vi "Process Depth.vi"(8 "Height":i32=480, 9 "Width":i32=640, 10 "Depth Format":u16(ring)=3 items=["11 Bit", "10 Bit", "11 Bit (Packed)", "10 Bit (Packed)"]) -> (3 "Depth Reshape Array":u16[][](array[numeric]))   [LabVIEW 2012]
panel:
  out "error out":errorcluster
  in  "error in":errorcluster
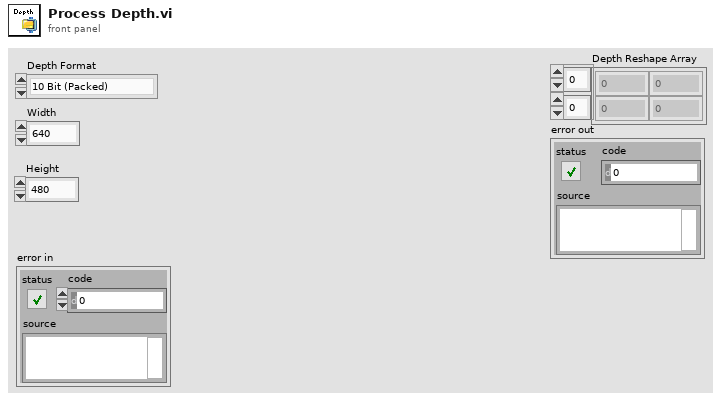
[diagram p1: front panel]
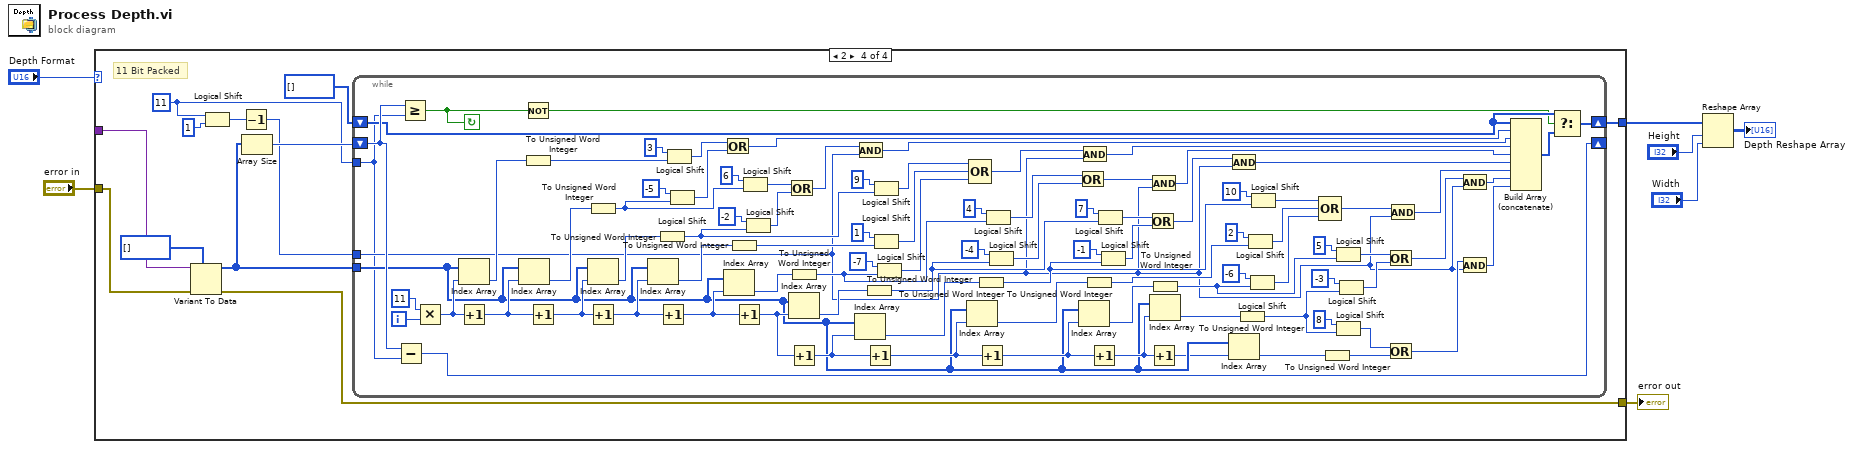
[diagram p0: block diagram]
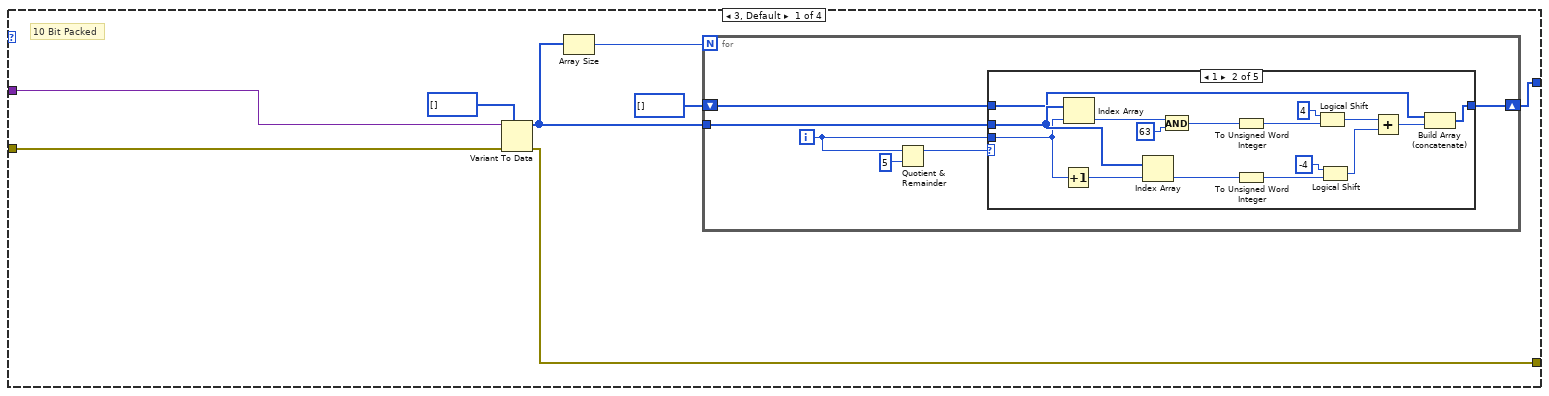
[diagram p2: hidden frame]
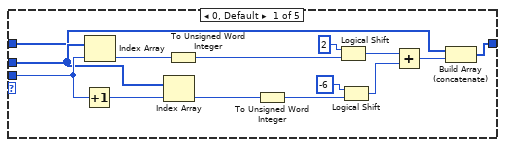
[diagram p3: hidden frame]
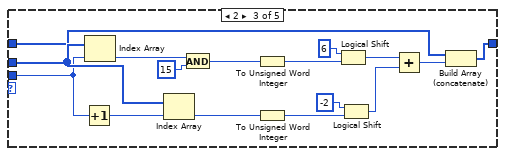
[diagram p4: hidden frame]
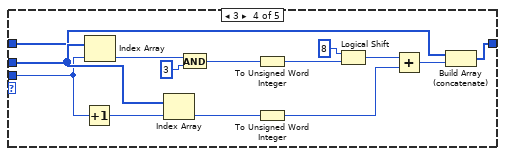
[diagram p5: hidden frame]
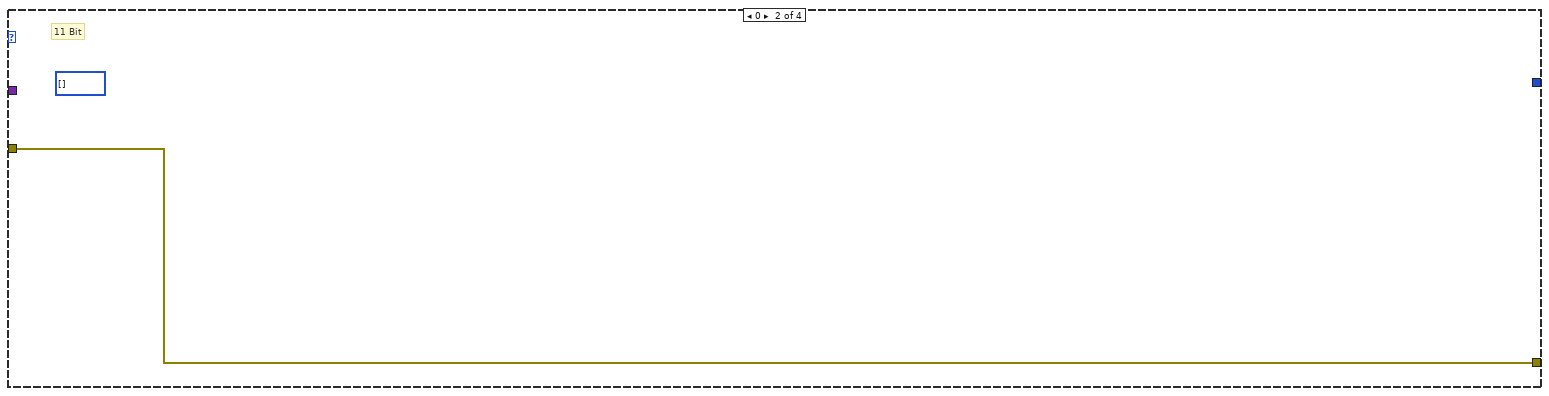
[diagram p7: hidden frame]
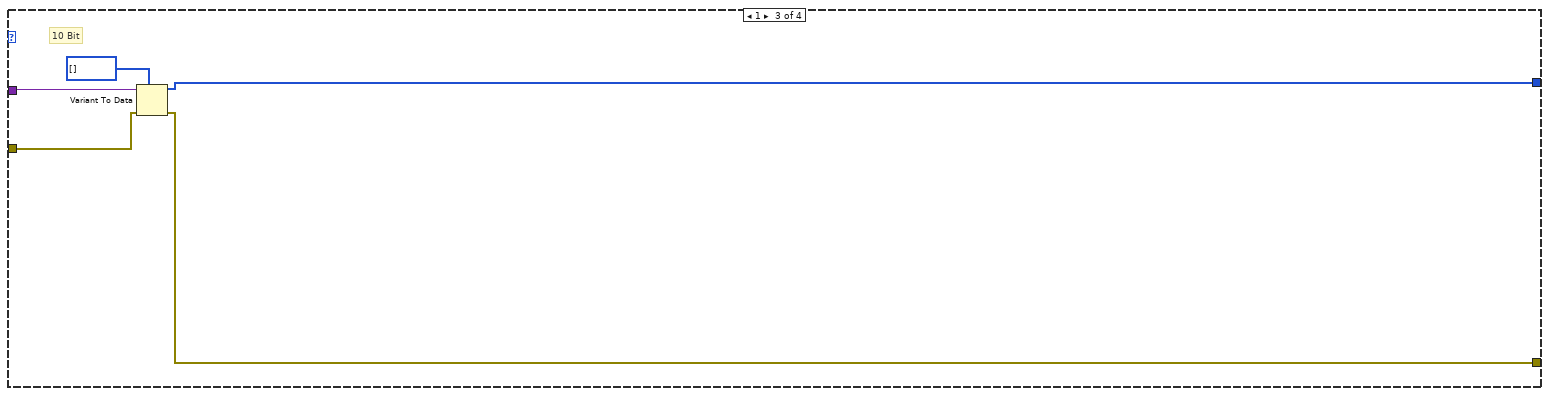
[diagram p8: hidden frame]
diagram:
  n1 = case shown="2" "Depth Format" {
    tunnel: [w14 w84 w87 w101] -> w6
    tunnel: _ -> [w12 w86 w88 w96]
    tunnel: "error in" -> [w11 w83 w91 w93]
    tunnel: [w9 w83 w90 w92] -> w1
    frame 3, Default {
      # "10 Bit Packed"
      n2 = Variant To Data(error in=w11, type=u8[] [] ("Packed Depth Array"), Variant=w12) -> (data=w8:u8[], error out=w9:errorcluster)
      n3 = Array Size(array=w8) -> (size(s)=w13:i32)
      n4 = for {
        N: w13 -> [_]
        tunnel: w8 -> [w19]
        shift-right: [w16] -> w14
        shift-left: u16[] [] -> [w17]
        i -> [w18]
        n5 = Quotient & Remainder(x=w18, y=5) -> (x-y*floor(x/y)=w20:i32)  [unwired: 1 out]
        n6 = case shown="1" w20 {
          tunnel: w19 -> [w33 w50 w66 w80 _]
          tunnel: w18 -> [w34 w49 w65 w79 _]
          tunnel: w17 -> [w31 w47 w61 w75 w82]
          tunnel: [w30 w48 w62 w76 w82] -> w16
          frame 0, Default {
            n7 = Increment(x=w34) -> (x+1=w35:i32)
            n8 = Index Array(array=w33, index=w34) -> (element=w28:u8)
            n9 = Index Array(array=w33, index=w35) -> (element=w22:u8)
            n10 = To Unsigned Word Integer(number=w28) -> (unsigned 16bit integer=w27:u16)
            n11 = To Unsigned Word Integer(number=w22) -> (unsigned 16bit integer=w23:u16)
            n12 = Logical Shift(y=u16 2 ("x"), x=w27) -> (x << y=w26:u16)
            n13 = Logical Shift(y=i16 -6, x=w23) -> (x << y=w24:u16)
            n14 = Add(x=w26, y=w24) -> (x+y=w29:u16)
            n15 = Build Array (concatenate)(w31, w29) -> (w30:u16[])
          }
          frame 1 {
            n16 = Increment(x=w49) -> (x+1=w51:i32)
            n17 = Index Array(array=w50, index=w49) -> (element=w45:u8)
            n18 = Index Array(array=w50, index=w51) -> (element=w36:u8)
            n19 = And(x=w45, y=u8 63) -> (x .and. y?=w43:u8)
            n20 = To Unsigned Word Integer(number=w43) -> (unsigned 16bit integer=w42:u16)
            n21 = To Unsigned Word Integer(number=w36) -> (unsigned 16bit integer=w37:u16)
            n22 = Logical Shift(y=i16 4, x=w42) -> (x << y=w40:u16)
            n23 = Logical Shift(y=i16 -4, x=w37) -> (x << y=w38:u16)
            n24 = Add(x=w40, y=w38) -> (x+y=w46:u16)
            n25 = Build Array (concatenate)(w47, w46) -> (w48:u16[])
          }
          frame 2 {
            n26 = Increment(x=w65) -> (x+1=w67:i32)
            n27 = Index Array(array=w66, index=w65) -> (element=w59:u8)
            n28 = Index Array(array=w66, index=w67) -> (element=w53:u8)
            n29 = And(x=w59, y=u8 15) -> (x .and. y?=w56:u8)
            n30 = To Unsigned Word Integer(number=w56) -> (unsigned 16bit integer=w57:u16)
            n31 = To Unsigned Word Integer(number=w53) -> (unsigned 16bit integer=w52:u16)
            n32 = Logical Shift(y=i16 6, x=w57) -> (x << y=w63:u16)
            n33 = Logical Shift(y=i16 -2, x=w52) -> (x << y=w55:u16)
            n34 = Add(x=w63, y=w55) -> (x+y=w60:u16)
            n35 = Build Array (concatenate)(w61, w60) -> (w62:u16[])
          }
          frame 3 {
            n36 = Increment(x=w79) -> (x+1=w81:i32)
            n37 = Index Array(array=w80, index=w79) -> (element=w73:u8)
            n38 = Index Array(array=w80, index=w81) -> (element=w69:u8)
            n39 = And(x=w73, y=u8 3) -> (x .and. y?=w71:u8)
            n40 = To Unsigned Word Integer(number=w71) -> (unsigned 16bit integer=w70:u16)
            n41 = To Unsigned Word Integer(number=w69) -> (unsigned 16bit integer=w68:u16)
            n42 = Logical Shift(y=i16 8, x=w70) -> (x << y=w77:u16)
            n43 = Add(x=w77, y=w68) -> (x+y=w74:u16)
            n44 = Build Array (concatenate)(w75, w74) -> (w76:u16[])
          }
          frame 4 {
          }
        }
      }
    }
    frame 0 {
      w85 = u16[] [] ("Packed Depth Array")
      # "11 Bit"
    }
    frame 1 {
      # "10 Bit"
      n45 = Variant To Data(error in=w91, type=u8[] [] ("Packed Depth Array"), Variant=w88) -> (data=w87:u8[], error out=w90:errorcluster)
    }
    frame 2 {
      w99 = 11 ("y")
      # "11 Bit Packed"
      n46 = Variant To Data(error in=w93, type=u8[] [] ("Packed Depth Array"), Variant=w96) -> (data=w94:u8[], error out=w92:errorcluster)
      n47 = Logical Shift(y=w99, x=1 ("y")) -> (x << y=w98:i32)
      n48 = Decrement(x=w98) -> (x-1=w97:i32)
      n49 = Array Size(array=w94) -> (size(s)=w103:i32)
      n50 = while {
        shift-right: [w197] -> _
        shift-left: w103 -> [w196]
        tunnel: w94 -> [w183]
        shift-right: [w107] -> w101
        shift-left: u16[] [] -> [w109]
        tunnel: w97 -> [w111]
        tunnel: w99 -> [w104]
        i -> [w195]
        stop <- w106 continue-if-true
        n51 = Subtract(x=w196, y=w104) -> (x-y=w197:i32)
        n52 = Greater Or Equal?(x=w196, y=w104) -> (x >= y?=w106:bool)
        n53 = Multiply(x=11, y=w195) -> (x*y=w193:i32)
        n54 = Index Array ("R0")(array=w183, index=w193) -> (element=w180:u8)
        n55 = Increment(x=w193) -> (x+1=w192:i32)
        n56 = Index Array ("R1")(array=w183, index=w192) -> (element=w178:u8)
        n57 = Not(x=w106) -> (.not. x?=w105:bool)
        n58 = To Unsigned Word Integer(number=w180) -> (unsigned 16bit integer=w181:u16)
        n59 = Increment(x=w192) -> (x+1=w191:i32)
        n60 = To Unsigned Word Integer(number=w178) -> (unsigned 16bit integer=w173:u16)
        n61 = Index Array ("R2")(array=w183, index=w191) -> (element=w171:u8)
        n62 = Increment(x=w191) -> (x+1=w190:i32)
        n63 = Index Array ("R3")(array=w183, index=w190) -> (element=w164:u8)
        n64 = To Unsigned Word Integer(number=w171) -> (unsigned 16bit integer=w167:u16)
        n65 = Increment(x=w190) -> (x+1=w189:i32)
        n66 = Logical Shift(y=i16 3, x=w181) -> (x << y=w175:u16)
        n67 = Logical Shift(y=i16 -5, x=w173) -> (x << y=w176:u16)
        n68 = Or(x=w175, y=w176) -> (x .or. y?=w174:u16)
        n69 = Index Array ("R4")(array=w183, index=w189) -> (element=w162:u8)
        n70 = To Unsigned Word Integer(number=w164) -> (unsigned 16bit integer=w165:u16)
        n71 = Increment(x=w189) -> (x+1=w188:i32)
        n72 = Logical Shift(y=i16 6, x=w173) -> (x << y=w168:u16)
        n73 = Logical Shift(y=i16 -2, x=w167) -> (x << y=w169:u16)
        n74 = Or(x=w168, y=w169) -> (x .or. y?=w123:u16)
        n75 = To Unsigned Word Integer(number=w162) -> (unsigned 16bit integer=w157:u16)
        n76 = Index Array ("R5")(array=w183, index=w188) -> (element=w155:u8)
        n77 = Increment(x=w188) -> (x+1=w187:i32)
        n78 = Index Array ("R6")(array=w183, index=w187) -> (element=w149:u8)
        n79 = And(x=w123, y=w111) -> (x .and. y?=w124:i32)
        n80 = To Unsigned Word Integer(number=w155) -> (unsigned 16bit integer=w151:u16)
        n81 = Increment(x=w187) -> (x+1=w186:i32)
        n82 = Logical Shift(y=i16 9, x=w167) -> (x << y=w160:u16)
        n83 = Logical Shift(y=i16 1, x=w165) -> (x << y=w159:u16)
        n84 = Logical Shift(y=i16 -7, x=w157) -> (x << y=w158:u16)
        n85 = Index Array ("R7")(array=w183, index=w186) -> (element=w143:u8)
        n86 = Compound Arithmetic op=OR(w160, w159, w158) -> (w122:u16)
        n87 = To Unsigned Word Integer(number=w149) -> (unsigned 16bit integer=w145:u16)
        n88 = Increment(x=w186) -> (x+1=w185:i32)
        n89 = Logical Shift(y=i16 4, x=w157) -> (x << y=w153:u16)
        n90 = Logical Shift(y=i16 -4, x=w151) -> (x << y=w152:u16)
        n91 = Or(x=w153, y=w152) -> (x .or. y?=w120:u16)
        n92 = Index Array ("R8")(array=w183, index=w185) -> (element=w140:u8)
        n93 = And(x=w122, y=w111) -> (x .and. y?=w121:i32)
        n94 = To Unsigned Word Integer(number=w143) -> (unsigned 16bit integer=w142:u16)
        n95 = Increment(x=w185) -> (x+1=w184:i32)
        n96 = Logical Shift(y=i16 7, x=w151) -> (x << y=w147:u16)
        n97 = Logical Shift(y=i16 -1, x=w145) -> (x << y=w146:u16)
        n98 = Or(x=w147, y=w146) -> (x .or. y?=w118:u16)
        n99 = And(x=w120, y=w111) -> (x .and. y?=w119:i32)
        n100 = Increment(x=w184) -> (x+1=w182:i32)
        n101 = To Unsigned Word Integer(number=w140) -> (unsigned 16bit integer=w135:u16)
        n102 = Index Array ("R9")(array=w183, index=w184) -> (element=w133:u8)
        n103 = And(x=w118, y=w111) -> (x .and. y?=w117:i32)
        n104 = Index Array ("R10")(array=w183, index=w182) -> (element=w125:u8)
        n105 = To Unsigned Word Integer(number=w133) -> (unsigned 16bit integer=w129:u16)
        n106 = Logical Shift(y=i16 2, x=w142) -> (x << y=w137:u16)
        n107 = Logical Shift(y=i16 -6, x=w135) -> (x << y=w136:u16)
        n108 = Logical Shift(y=i16 10, x=w145) -> (x << y=w138:u16)
        n109 = Compound Arithmetic op=OR(w138, w137, w136) -> (w116:u16)
        n110 = To Unsigned Word Integer(number=w125) -> (unsigned 16bit integer=w126:u16)
        n111 = Logical Shift(y=i16 5, x=w135) -> (x << y=w131:u16)
        n112 = Logical Shift(y=i16 8, x=w129) -> (x << y=w127:u16)
        n113 = Logical Shift(y=i16 -3, x=w129) -> (x << y=w130:u16)
        n114 = Or(x=w131, y=w130) -> (x .or. y?=w114:u16)
        n115 = Or(x=w127, y=w126) -> (x .or. y?=w112:u16)
        n116 = And(x=w116, y=w111) -> (x .and. y?=w115:i32)
        n117 = And(x=w114, y=w111) -> (x .and. y?=w113:i32)
        n118 = And(x=w112, y=w111) -> (x .and. y?=w110:i32)
        n119 = Build Array (concatenate)(w109, w174, w124, w121, w119, w117, w115, w113, w110) -> (w108:i32[])
        n120 = Select(t=w109, s=w105, f=w108) -> (s? t:f=w107:i32[])
      }
    }
  }
  "error out" <- w1
  n121 = Reshape Array(w6, "Height", "Width") -> (→"Depth Reshape Array":i32[][])
